vi "29-Equipment Requests Time Value from Host.vi"(8 "error in":errorcluster) -> (0 "error out":errorcluster, 2 "Timeout?":bool, 3 "Time":string)   [LabVIEW 2020, in "SECS Scenarios.lvlib" / "Scenarios Class.lvclass"]
uses:
  Scenarios Class.lvclass
  29-Equipment Requests Time Value from Host.ctl
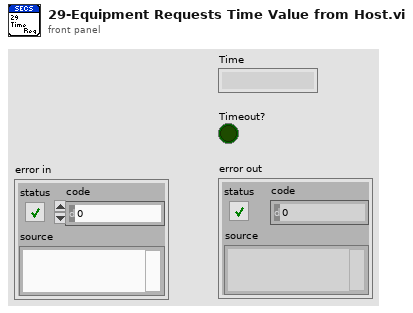
[diagram p1: front panel]
types:
  T1 = typedef "SECS Scenarios.lvlib/Scenarios Class.lvclass/29-Equipment Requests Time Value from Host.ctl" = cluster{"Reply Notifier":refnum<notifier>}
  T2 = typedef "SECS Scenarios.lvlib/Scenarios Class.lvclass/Request Refnum.ctl" = cluster{"11-Alarm Management":refnum<user-event>, "07-Event Report From Equipment":refnum<user-event>, "14-Process Program Creating Editing or Deleting":refnum<user-event>, "21-Material Movement":refnum<user-event>, "23-Equipment Sends Information to Host":refnum<user-event>, "24-Host Accepts On-Line Request from Equipment":refnum<user-event>, "25-Host Refuses On-Line Request":refnum<user-event>, "29-Equipment Requests Time Value from Host":refnum<user-event>, "33-Update Trace Data":refnum<user-event>}
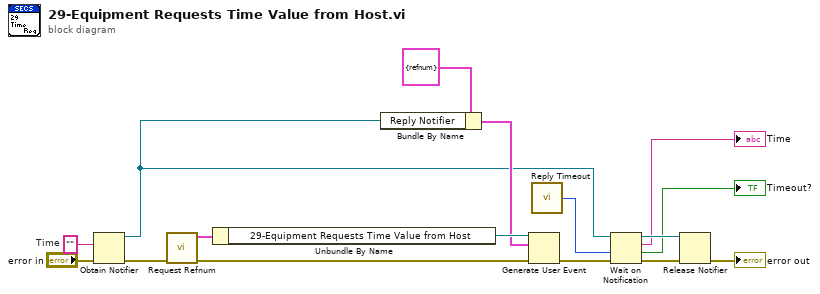
[diagram p0: block diagram]
diagram:
  w13 = ""  # Time
  n1 = Obtain Notifier(notification data type=w13, error in (no error)="error in") -> (notifier out=w5:refnum<notifier>, error out=w11:errorcluster)  [unwired: 2 in, 1 out]
  n2 = call "Request Refnum.vi"("error in"=w11) -> ("error out"=w15:errorcluster, "Request Refnum"=w16:T2)  [unwired: 9 in]
  n3 = Unbundle By Name(w16) -> ("29-Equipment Requests Time Value from Host"=w14:refnum<user-event>)
  n4 = Bundle By Name(cluster=T1 {"Reply Notifier"=refnum} ("29-Equipment Requests Time Value from Host"), "Reply Notifier"=w5) -> (w9:T1)
  n5 = Generate User Event(user event=w14, event data cluster=w9, error in=w15) -> (error out=w6:errorcluster)  [unwired: 1 in, 1 out]
  n6 = call "Reply Timeout.vi"() -> ("Reply Timeout"=w4:i32)
  n7 = Wait on Notification(notifier=w5, timeout in ms (-1)=w4, error in (no error)=w6) -> (notifier out=w8:refnum<notifier>, notification=→"Time":string, timed out?=→"Timeout?":bool, error out=w7:errorcluster)  [unwired: 1 in]
  n8 = Release Notifier(notifier=w8, error in (no error)=w7) -> (error out=→"error out":errorcluster)  [unwired: 1 in, 2 out]
